vi "Monitor System Resources.vi"(8 "error in (no error)":errorcluster, 11 "Number of CPU Cores":u64) -> (0 "error out":errorcluster, 3 "System Resources":dbl[](array[numeric]))   [LabVIEW 2027, in "System Monitor Engine.lvlib"]
uses:
  System Monitor Engine.lvlib
  <resource>/objmgr/nisysapi.rc
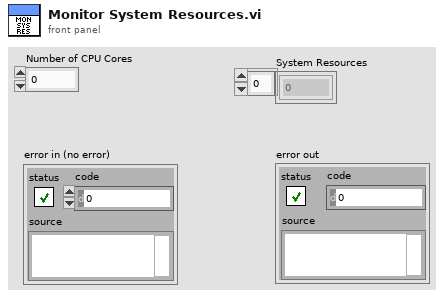
[diagram p1: front panel]
types:
  T1 = typedef "NI_Real-Time Target Support.lvlib/RT CPU Load.ctl" = cluster{"Total (%)":dbl, "Time Critical (%)":dbl, "Timed Structures (%)":dbl, "High (%)":dbl, "Above Normal (%)":dbl, "Normal (%)":dbl, "Background (%)":dbl, "Idle (%)":dbl, "ISR (%)":dbl}
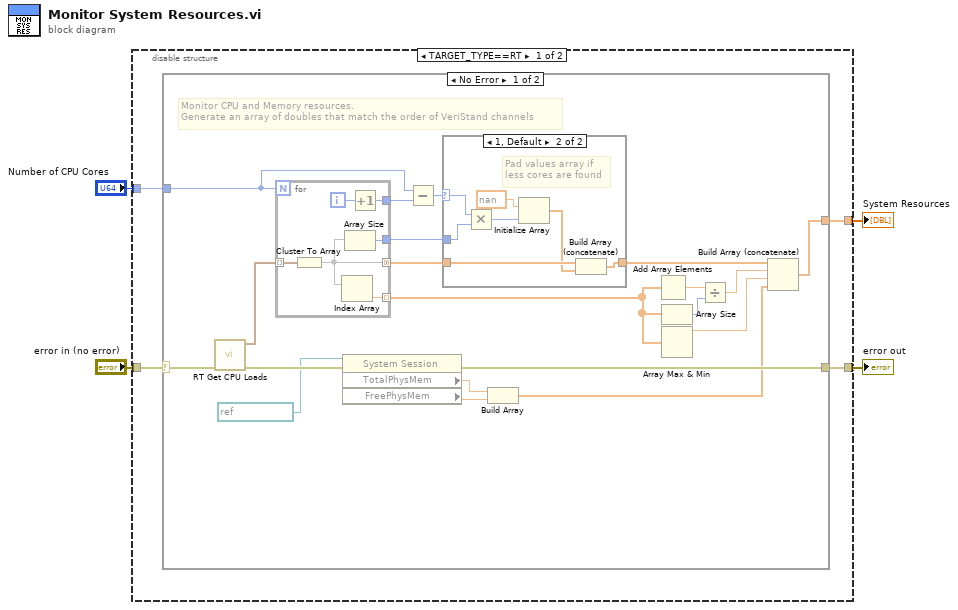
[diagram p0: block diagram]
diagram:
  n1 = disable-structure shown="TARGET_TYPE==RT" {
    disable-tunnel: "Number of CPU Cores" -> [w8 _]
    disable-tunnel: [w6 _] -> w3
    disable-tunnel: "error in (no error)" -> [w7 _]
    disable-tunnel: [w5 _] -> w1
    frame condition #0 {
      n2 = case shown="No Error" w7 {
        selector: w7 -> [w25 w43]
        tunnel: w8 -> [w17 _]
        tunnel: [w26 w43] -> w6
        tunnel: [w22 _] -> w5
        frame No Error {
          # "Monitor CPU and Memory resources.\nGenerate an array of doubles that match the order of VeriStand channels"
          n3 = call <vilib>:"RT Get CPU Loads.vi"("error in (no error)"=w25) -> ("error out"=w27:errorcluster, "CPU loads"=w28:T1[])  [unwired: 9 in]
          n4 = for {
            N: w17 -> [_]
            tunnel: w28 -> [w42] mode=indexing
            tunnel: [w38] -> w19 mode=concatenating
            tunnel: [w39] -> w16
            tunnel: [w40] -> w20
            tunnel: [w37] -> w9 mode=indexing
            i -> [w41]
            n5 = Cluster To Array(cluster=w42) -> (array=w38:dbl[])
            n6 = Index Array(array=w38) -> (element=w37:dbl)  [unwired: 1 in]
            n7 = Array Size(array=w38) -> (size(s)=w40:i32)
            n8 = Increment(x=w41) -> (x+1=w39:i32)
          }
          n9 = property class="System Session"(reference=refnum<k21> "localhost" ("System Configuration"), error in=w27) -> (error out=w26:errorcluster, "TotalPhysMem"=w24:dbl, "FreePhysMem"=w23:dbl)  [unwired: 1 out]
          n10 = Subtract(x=w17, y=w16) -> (x-y=w18:u64)
          n11 = case shown="1, Default" w18 {
            selector: w18 -> [_ w35]
            tunnel: w20 -> [_ w36]
            tunnel: w19 -> [w29 w33]
            tunnel: [w29 w32] -> w11
            frame 0 {
            }
            frame 1, Default {
              # "Pad values array if\nless cores are found"
              n12 = Multiply(x=w35, y=w36) -> (x*y=w34:u64)
              n13 = Initialize Array(nan, w34) -> (w31:dbl[])
              n14 = Build Array (concatenate)(w33, w31) -> (w32:dbl[])
            }
          }
          n15 = Build Array(w24, w23) -> (w14:dbl[])
          n16 = Add Array Elements(numeric array=w9) -> (sum=w10:dbl)
          n17 = Array Size(array=w9) -> (size(s)=w15:i32)
          n18 = Array Max & Min(array=w9) -> (max value=w12:dbl)  [unwired: 3 out]
          n19 = Divide(x=w10, y=w15) -> (x/y=w13:dbl)
          n20 = Build Array (concatenate)(w11, w13, w12, w14) -> (w22:dbl[])
        }
        frame Error {
        }
      }
    }
    frame condition #1 (active) {
    }
  }
  "error out" <- w3
  "System Resources" <- w1
